vi "DriveDashModule.vi"(11 "Module":i32) -> (0 "SpinAbsPosDeg":dbl, 1 "TravMotDmd":dbl, 2 "TravSpeedFPS":dbl, 3 "TravSpdDmdFPS":dbl, 5 "TravDistFt":dbl, 8 "Prefix":string)   [LabVIEW 2023]
doc: "Network for Drive\n\nInputs:\n -- Error in -- Error cluster -- propagated error input\n\nOutputs:\n -- Error out -- Error cluster -- progated error output"
uses:
  <vilib>/Rock Robotics/Network Tables/NT Read Number.vi
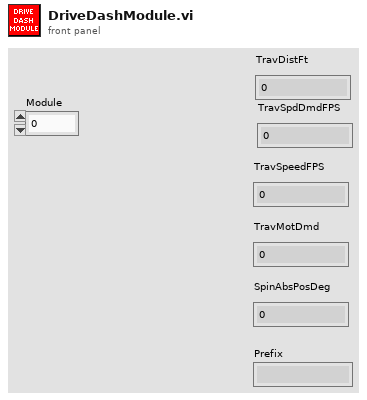
[diagram p1: front panel]
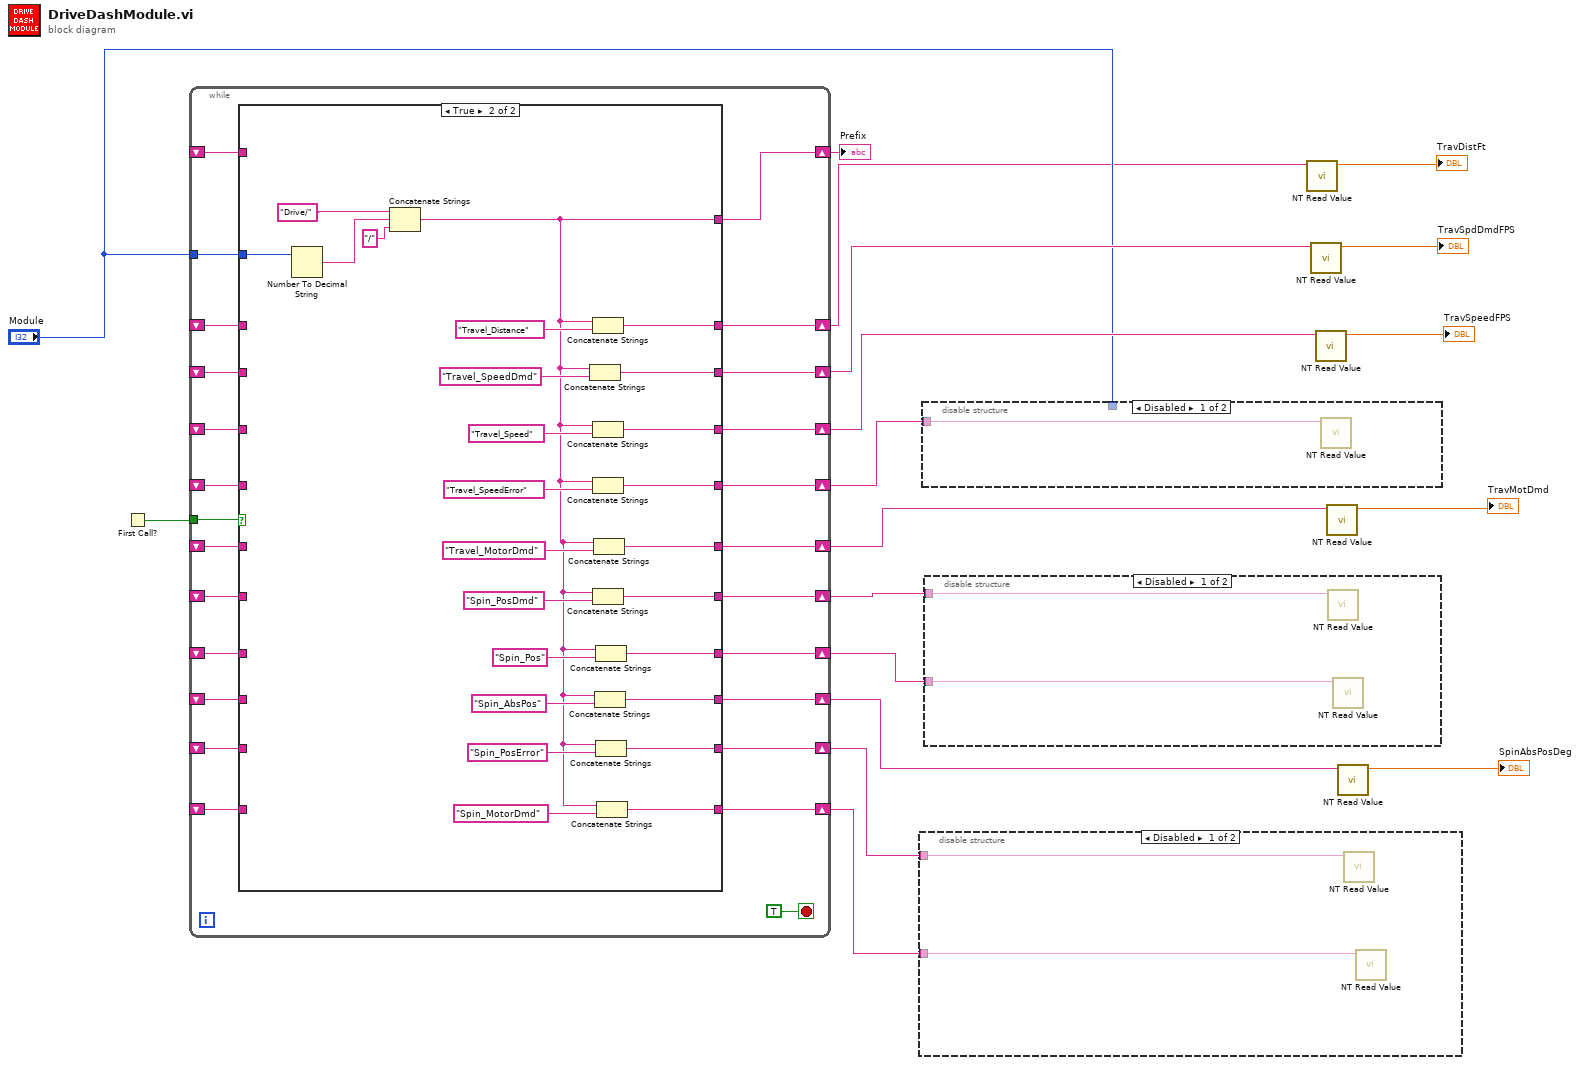
[diagram p0: block diagram]
diagram:
  n1 = First Call?() -> (First Call?: T/F=w18:bool)
  n2 = while {
    tunnel: w18 -> [w42]
    tunnel: "Module" -> [w41]
    shift-right: [w40] -> w17
    shift-left: _ -> [w31]
    shift-right: [w39] -> w16
    shift-left: _ -> [w30]
    shift-right: [w38] -> w15
    shift-left: _ -> [w28]
    shift-right: [w37] -> w14
    shift-left: _ -> [w29]
    shift-right: [w36] -> w13
    shift-left: _ -> [w27]
    shift-right: [w35] -> w12
    shift-left: _ -> [w26]
    shift-right: [w34] -> w11
    shift-left: _ -> [w25]
    shift-right: [w33] -> w10
    shift-left: _ -> [w24]
    shift-right: [w32] -> w9
    shift-left: _ -> [w23]
    shift-right: [w22] -> w7
    shift-left: _ -> [w21]
    shift-right: [w20] -> w1
    shift-left: _ -> [w19]
    stop <- TRUE stop-if-true
    n3 = case shown="True" w42 {
      tunnel: w41 -> [_ w78]
      tunnel: [w54 w66] -> w40
      tunnel: [w53 w65] -> w39
      tunnel: [w51 w64] -> w38
      tunnel: [w52 w63] -> w37
      tunnel: [w50 w62] -> w36
      tunnel: [w49 w61] -> w35
      tunnel: [w48 w60] -> w34
      tunnel: [w47 w59] -> w33
      tunnel: [w46 w58] -> w32
      tunnel: w31 -> [w54 _]
      tunnel: w30 -> [w53 _]
      tunnel: w29 -> [w52 _]
      tunnel: w28 -> [w51 _]
      tunnel: w27 -> [w50 _]
      tunnel: w26 -> [w49 _]
      tunnel: w25 -> [w48 _]
      tunnel: w24 -> [w47 _]
      tunnel: w23 -> [w46 _]
      tunnel: [w45 w56] -> w22
      tunnel: w21 -> [w45 _]
      tunnel: [w44 w55] -> w20
      tunnel: w19 -> [w44 _]
      frame False {
      }
      frame True {
        n4 = Number To Decimal String(number=w78) -> (decimal integer string=w77:string)  [unwired: 1 in]
        n5 = Concatenate Strings("Drive/", w77, "/" ("string")) -> (w55:string)
        n6 = Concatenate Strings(w55, "Travel_SpeedDmd" ("string")) -> (w66:string)
        n7 = Concatenate Strings(w55, "Travel_Distance" ("string")) -> (w56:string)
        n8 = Concatenate Strings(w55, "Travel_Speed" ("string")) -> (w65:string)
        n9 = Concatenate Strings(w55, "Travel_SpeedError" ("string")) -> (w64:string)
        n10 = Concatenate Strings(w55, "Spin_PosDmd" ("string")) -> (w62:string)
        n11 = Concatenate Strings(w55, "Travel_MotorDmd" ("string")) -> (w63:string)
        n12 = Concatenate Strings(w55, "Spin_AbsPos" ("string")) -> (w60:string)
        n13 = Concatenate Strings(w55, "Spin_Pos" ("string")) -> (w61:string)
        n14 = Concatenate Strings(w55, "Spin_PosError" ("string")) -> (w59:string)
        n15 = Concatenate Strings(w55, "Spin_MotorDmd" ("string")) -> (w58:string)
      }
    }
  }
  "Prefix" <- w1
  n16 = disable-structure shown="Disabled" {
    disable-tunnel: w10 -> [w81 _]
    disable-tunnel: w9 -> [w80 _]
    frame Disabled {
      n17 = call-poly <vilib>:"NT Read Value.vi"("name"=w81) -> ()  [unwired: 8 in, 3 out]
      n18 = call-poly <vilib>:"NT Read Value.vi"("name"=w80) -> ()  [unwired: 8 in, 3 out]
    }
    frame Enabled {
    }
  }
  n19 = disable-structure shown="Disabled" {
    disable-tunnel: w15 -> [w82 _]
    disable-tunnel: "Module" -> [_ _]
    frame Disabled {
      n20 = call-poly <vilib>:"NT Read Value.vi"("name"=w82) -> ()  [unwired: 8 in, 3 out]
    }
    frame Enabled {
    }
  }
  n21 = disable-structure shown="Disabled" {
    disable-tunnel: w13 -> [w84 _]
    disable-tunnel: w12 -> [w83 _]
    frame Disabled {
      n22 = call-poly <vilib>:"NT Read Value.vi"("name"=w84) -> ()  [unwired: 8 in, 3 out]
      n23 = call-poly <vilib>:"NT Read Value.vi"("name"=w83) -> ()  [unwired: 8 in, 3 out]
    }
    frame Enabled {
    }
  }
  n24 = call-poly <vilib>:"NT Read Value.vi"("name"=w7) -> ("value"=→"TravDistFt":dbl)  [unwired: 8 in, 2 out]
  n25 = call-poly <vilib>:"NT Read Value.vi"("name"=w17) -> ("value"=→"TravSpdDmdFPS":dbl)  [unwired: 8 in, 2 out]
  n26 = call-poly <vilib>:"NT Read Value.vi"("name"=w16) -> ("value"=→"TravSpeedFPS":dbl)  [unwired: 8 in, 2 out]
  n27 = call-poly <vilib>:"NT Read Value.vi"("name"=w14) -> ("value"=→"TravMotDmd":dbl)  [unwired: 8 in, 2 out]
  n28 = call-poly <vilib>:"NT Read Value.vi"("name"=w11) -> ("value"=→"SpinAbsPosDeg":dbl)  [unwired: 8 in, 2 out]
